vi "Volatus GUI Editor.vi"() -> ()   [LabVIEW 2020, in "VolatusGUIEditor.lvlib"]
uses:
  VolatusGUIEditor.lvlib
  UI Refs.ctl
  Editor/Editor.lvclass
panel:
  in  "Elements":string(tree)
  out "Description":string
  out "Picture":picture
  # "Available Elements"
  # "Preview"
  # "Select a control in a GUI to edit its properties."
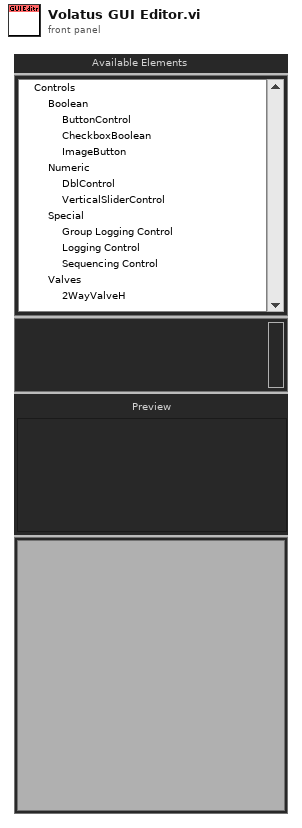
[diagram p1: front panel]
types:
  T1 = typedef "VolatusGUIEditor.lvlib/UI Refs.ctl" = cluster{"Elements":refnum<vi>, "Description":refnum<vi>, "Picture":refnum<vi>, "Panel":refnum<vi>}
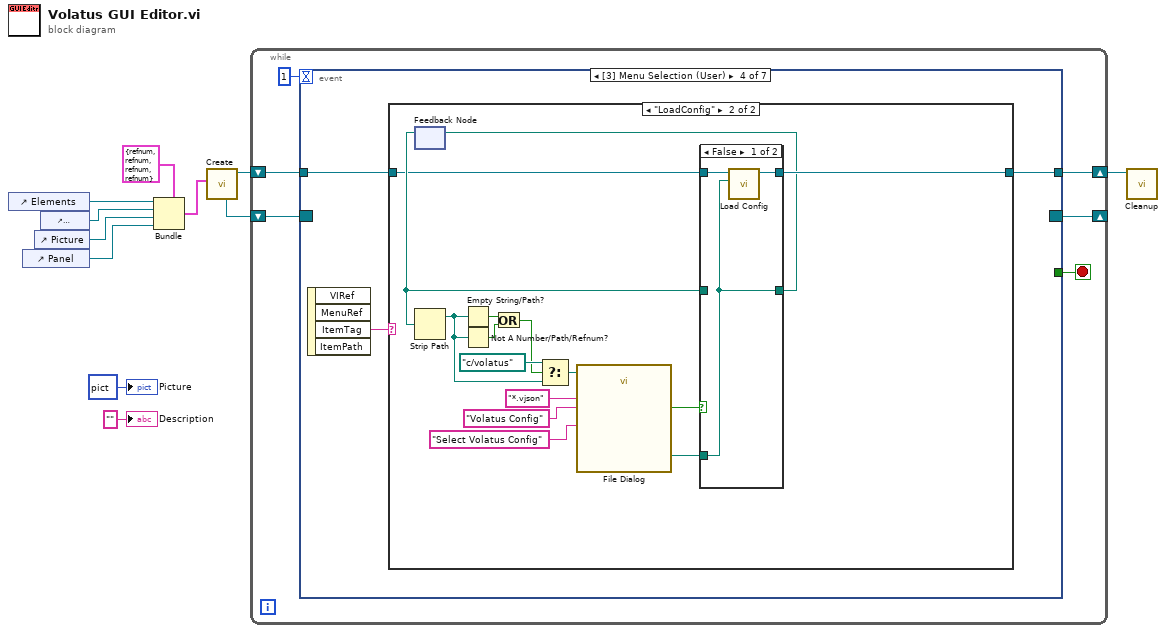
[diagram p0: block diagram]
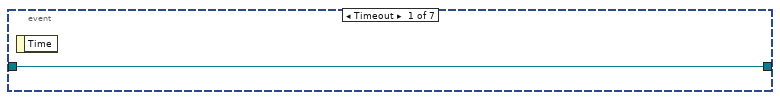
[diagram p2: hidden frame]
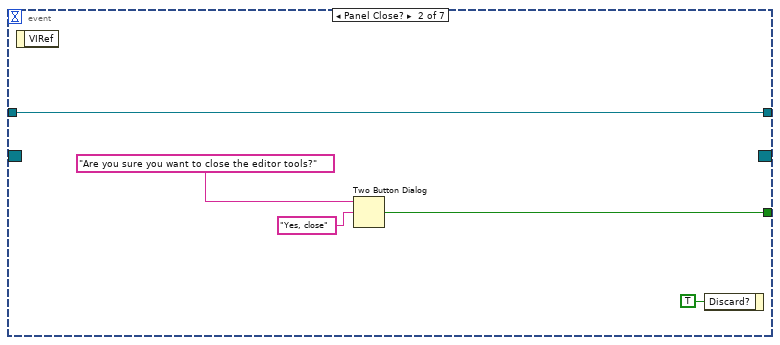
[diagram p3: hidden frame]
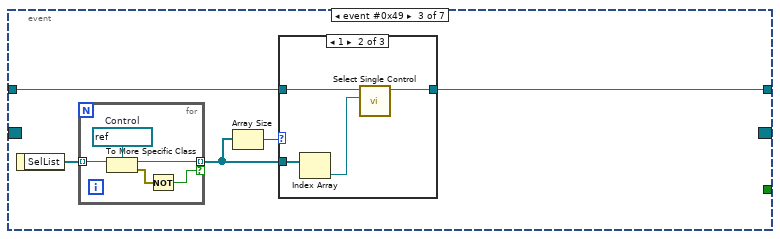
[diagram p4: hidden frame]
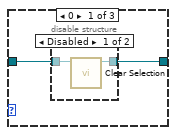
[diagram p5: hidden frame]
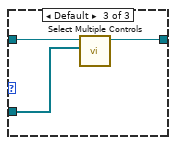
[diagram p7: hidden frame]
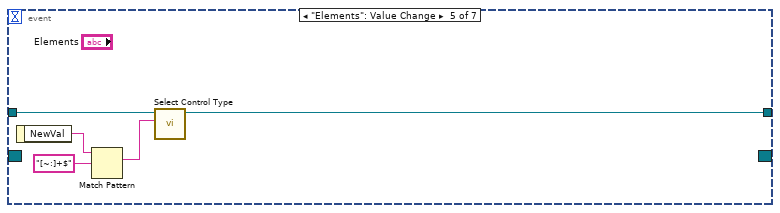
[diagram p10: hidden frame]
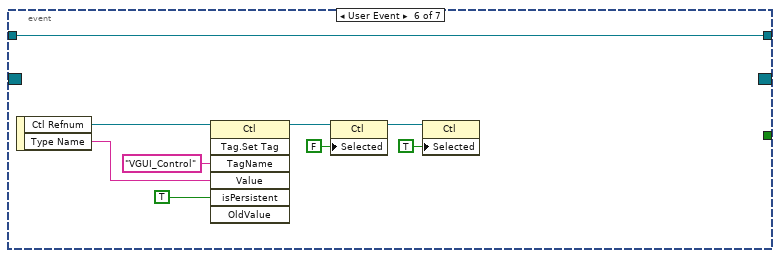
[diagram p11: hidden frame]
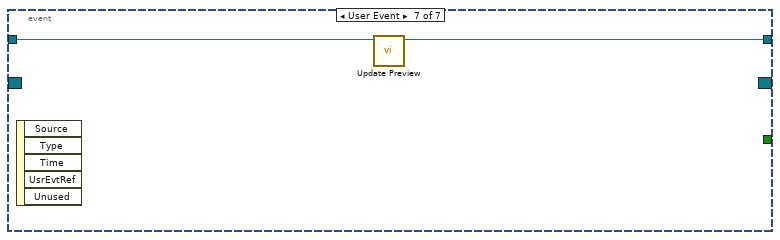
[diagram p12: hidden frame]
diagram:
  n1 = control-ref of="Elements"() -> (w9:refnum<vi>)
  n2 = control-ref of="Panel"() -> (w6:refnum<vi>)
  n3 = control-ref of="Picture"() -> (w7:refnum<vi>)
  n4 = control-ref of="Description"() -> (w8:refnum<vi>)
  n5 = Bundle(cluster=T1 {"Elements"=refnum, "Description"=refnum, "Picture"=refnum, "Panel"=refnum} ("UI Refs"), "Elements"=w9, "Description"=w8, "Picture"=w7, "Panel"=w6) -> (w4:T1)
  n6 = call "Create.vi"("UI Refs"=w4) -> ("Editor out"=w11:refnum<class "Editor.lvclass">, "Event Reg"=w3:refnum<event-registration>)  [unwired: 8 in, 1 out]
  n7 = while {
    shift-right: [w15] -> w10
    shift-left: w11 -> [w16]
    shift-right: [w12] -> _
    shift-left: w3 -> [w13]
    stop <- w14 stop-if-true
    n8 = event shown="[3] Menu Selection (User)" {
      selector: w13 -> [_ _ _ _ _ _ _]
      dyn-events: [_ _ _ _ _ _ _] -> w12
      timeout: 1 -> [_ _ _ _ _ _ _]
      tunnel: w16 -> [w18 w23 w27 w48 w74 w83 w85]
      tunnel: [w18 w23 w26 w46 w71 w83 w84] -> w15
      tunnel: [_ w19 _ _ _ _ _] -> w14
      event Timeout {
        n9 = event-data() -> ()  [unwired: 1 in, 1 out]
      }
      event Panel Close? {
        n10 = event-data() -> ()  [unwired: 1 in, 1 out]
        n11 = Two Button Dialog(message="Are you sure you want to close the editor tools?", 2:"Yes, close" ("T button name (\"OK\")")) -> (T button?=w19:bool)  [unwired: 1 in]
        n12 = event-data("Discard?"=TRUE) -> ()  [unwired: 1 in, 1 out]
      }
      event event #0x49 {
        n13 = event-data() -> ("SelList"=w25:refnum<vi>[])  [unwired: 1 in]
        n14 = for {
          tunnel: w25 -> [w32] mode=indexing
          tunnel: [w31] -> w24 mode=indexing if=w29
          w33 = refnum<vi> refnum  # Control
          n15 = To More Specific Class(target class=w33, reference=w32) -> (specific class reference=w31:refnum<vi>, error out=w30:errorcluster)  [unwired: 1 in]
          n16 = Not(x=w30) -> (.not. x?=w29:bool)
        }
        n17 = Array Size(array=w24) -> (size(s)=w28:i32)
        n18 = case shown="1" w28 {
          tunnel: w27 -> [w35 w42 w45]
          tunnel: [w34 w41 w44] -> w26
          tunnel: w24 -> [_ w40 w43]
          frame 0 {
            n19 = disable-structure shown="Disabled" {
              disable-tunnel: w35 -> [w37 w38]
              disable-tunnel: [w36 w38] -> w34
              frame Disabled {
                n20 = call "Clear Selection.vi"("Editor in"=w37) -> ("Editor out"=w36:refnum<class "Editor.lvclass">)  [unwired: 9 in, 1 out]
              }
              frame Enabled {
              }
            }
          }
          frame 1 {
            n21 = Index Array(array=w40) -> (element=w39:refnum<vi>)  [unwired: 1 in]
            n22 = call "Select Single Control.vi"("Ctl Refnum"=w39, "Editor in"=w42) -> ("Editor out"=w41:refnum<class "Editor.lvclass">)  [unwired: 8 in, 1 out]
          }
          frame Default {
            n23 = call "Select Multiple Controls.vi"("Controls"=w43, "Editor in"=w45) -> ("Editor out"=w44:refnum<class "Editor.lvclass">)  [unwired: 8 in, 1 out]
          }
        }
      }
      event Menu Selection (User) {
        n24 = event-data() -> ("ItemTag"=w47:string)  [unwired: 1 in, 3 out]
        n25 = case shown="\"LoadConfig\"" w47 {
          tunnel: w48 -> [w49 w52]
          tunnel: [w49 w51] -> w46
          frame Default {
          }
          frame "LoadConfig" {
            n26 = feedback #1() -> (w53:path)  [unwired: 1 in]
            n27 = Strip Path(path=w53) -> (stripped path=w56:path)  [unwired: 1 out]
            n28 = Empty String/Path?(string/path=w56) -> (empty?=w60:bool)
            n29 = Not A Number/Path/Refnum?(number/path/refnum=w56) -> (NaN/Path/Refnum?=w59:bool)
            n30 = Or(x=w60, y=w59) -> (x .or. y?=w58:bool)
            n31 = Select(t=path "c:/volatus", s=w58, f=w56) -> (s? t:f=w57:path)
            n32 = call "File Dialog"("start path"=w57, "prompt"="Select Volatus Config", "pattern (all files)"="*.vjson", "pattern label"="Volatus Config") -> ("selected path"=w54:path, "cancelled"=w55:bool)  [unwired: 8 in, 2 out]
            n33 = case shown="False" w55 {
              tunnel: w54 -> [w66 _]
              tunnel: w53 -> [_ w68]
              tunnel: w52 -> [w67 w69]
              tunnel: [w65 w69] -> w51
              tunnel: [w66 w68] -> w50
              frame False {
                n34 = call "Load Config.vi"("Config Path"=w66, "Editor in"=w67) -> ("Editor out"=w65:refnum<class "Editor.lvclass">)  [unwired: 8 in, 1 out]
              }
              frame True {
              }
            }
            n35 = feedback-in #1(w50) -> ()
          }
        }
      }
      event "Elements": Value Change {
        n36 = event-data() -> ("NewVal"=w73:string)  [unwired: 1 in]
        n37 = Match Pattern(string=w73, regular expression="[~:]+$") -> (match substring=w70:string)  [unwired: 1 in, 3 out]
        n38 = call "Select Control Type.vi"("Control Type"=w70, "Editor in"=w74) -> ("Editor out"=w71:refnum<class "Editor.lvclass">)  [unwired: 8 in, 1 out]
      }
      event User Event {
        n39 = event-data() -> ("Ctl Refnum"=w79:refnum<vi>, "Type Name"=w82:string)  [unwired: 1 in]
        n40 = invoke class="Ctl" method="Tag.Set Tag"(reference=w79, "TagName"="VGUI_Control" ("Tag Name"), "Value"=w82, "isPersistent"=TRUE ("Is Persistent?")) -> (reference out=w78:refnum<vi>)  [unwired: 3 in, 6 out]
        n41 = property class="Ctl"(reference=w78, "Selected"=FALSE) -> (reference out=w76:refnum<vi>)  [unwired: 1 in, 1 out]
        n42 = property class="Ctl"(reference=w76, "Selected"=TRUE) -> ()  [unwired: 1 in, 2 out]
      }
      event User Event {
        n43 = event-data() -> ()  [unwired: 1 in, 5 out]
        n44 = call "Update Preview.vi"("Editor in"=w85) -> ("Editor out"=w84:refnum<class "Editor.lvclass">)  [unwired: 9 in, 1 out]
      }
    }
  }
  n45 = call "Cleanup.vi"("Editor in"=w10) -> ()  [unwired: 10 in, 1 out]
  "Picture" <- picture data[5B] ("Picture")
  "Description" <- "" ("Description")
